vi "TCP IP Read Tester.vi"() -> ()   [LabVIEW 2015]
uses:
  Controls/QMH Fundamentals - Message Cluster.ctl
panel:
  in  "Test Read String":bool
  out "JSON Message":string="{\"PhoenixMsg\": {\n    \"Partition\" : \"EMP\",\n    \"Message\" : \"MSG\",\n    \"EnergyChannelId\" : 1,\n    \"IsActivated\" : True,\n    \"StopReason\" : 3,\n    \"Mode\" : 1,\n    \"PowerLevel\" : 32,\n}}"
  in  "Read":bool
  out "Cluster":T1
  out "Array":T2(array[cluster])
  in  "Fornax Executable Path":path=path "C:/Program Files (x86)/Medtronic/Fornax/x86/Fornax.exe"
  in  "error in (no error)":errorcluster
  out "Bipolar - Mode":string
  out "Bipolar - Power":string
  out "Mono2 Coag - Mode":string
  out "Mono2 Coag - Power":string
  out "Mono2 Cut - Mode":string
  out "Mono2 Cut - Power":string
  out "Mono1 Coag - Mode":string
  out "Mono1 Coag - Power":string
  out "Mono1 Cut - Mode":string
  out "Mono1 Cut - Power":string
  in  "Read String":string
  in  "stop":bool
  # "Mono1"
  # "Mono2"
  # "Bipolar"
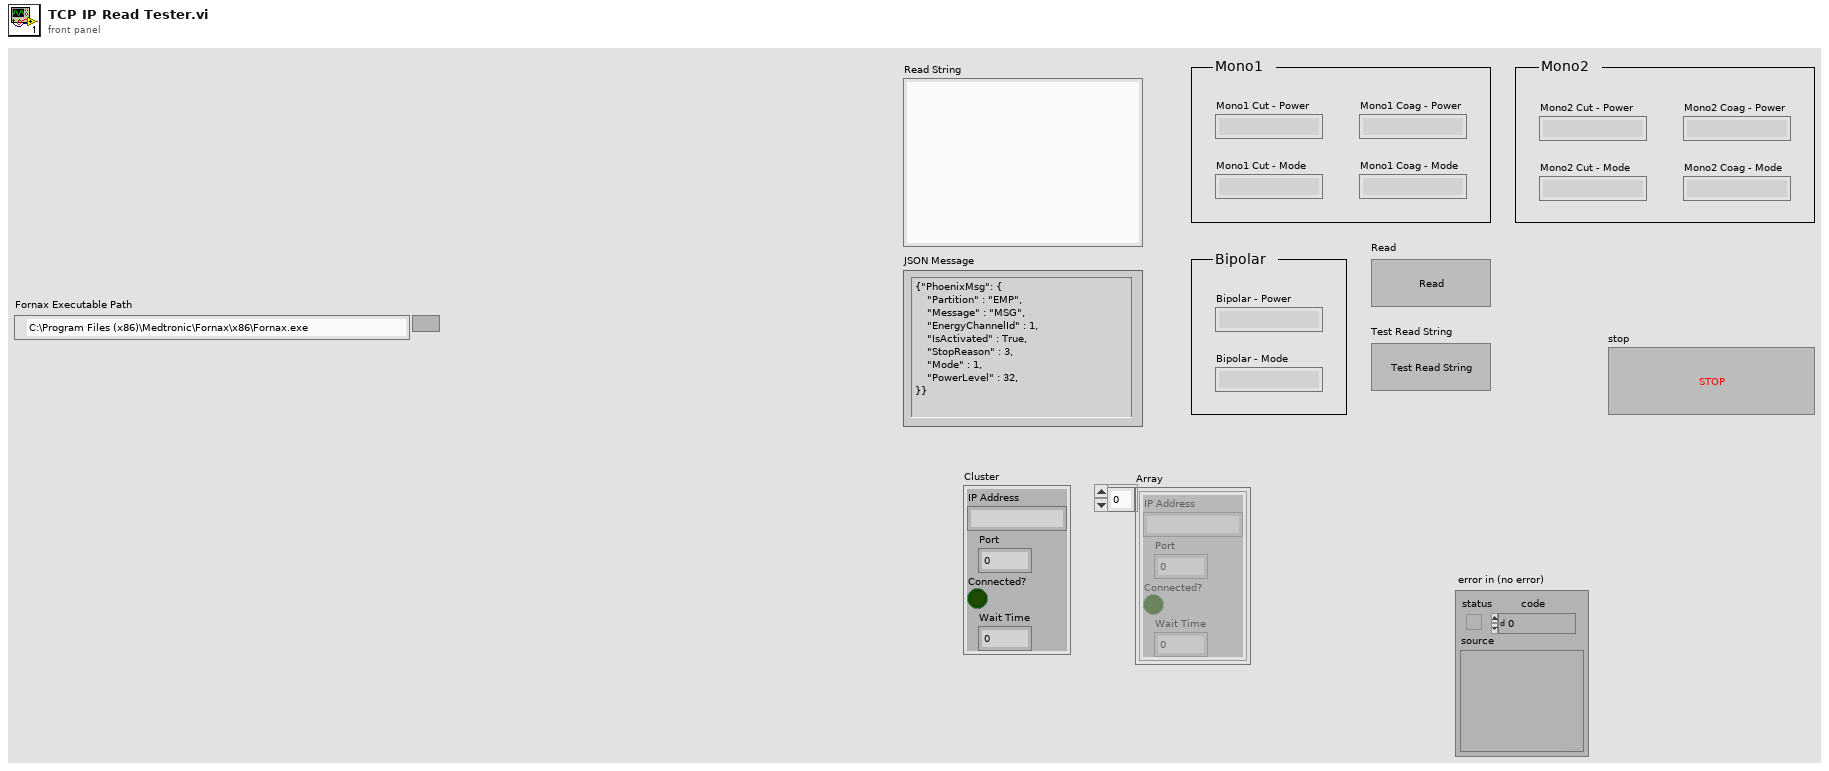
[diagram p1: front panel]
types:
  T1 = cluster{"IP Address":string, "Port":u16, "Connected?":bool, "Wait Time":dbl}
  T2 = cluster{"IP Address":string, "Port":u16, "Connected?":bool, "Wait Time":dbl}[]
  T3 = typedef "QMH Fundamentals - Message Cluster.ctl" = cluster{"Message":string, "Message Data":variant}
  T4 = cluster{"Mono1 Cut - Power":refnum<vi>, "Mono1 Cut - Mode":refnum<vi>, "Mono1 Coag - Power":refnum<vi>, "Mono1 Coag - Mode":refnum<vi>, "Mono2 Coag - Power":refnum<vi>, "Mono2 Coag - Mode":refnum<vi>, "Mono2 Cut - Power":refnum<vi>, "Mono2 Cut - Mode":refnum<vi>, "Bipolar - Power":refnum<vi>, "Bipolar - Mode":refnum<vi>}
  T5 = cluster{"Mono1 Cut Enum":refnum<vi>, "Mono1 - Cut Power":refnum<vi>, "Mono1 Coag Enum":refnum<vi>, "Mono1 - Coag Power":refnum<vi>, "Mono2 Cut Enum":refnum<vi>, "Mono2 - Cut Power":refnum<vi>, "Mono2 Coag Enum":refnum<vi>, "Mono2 - Coag Power":refnum<vi>, "Bipolar Enum":refnum<vi>, "Mono1 - Bipolar Power":refnum<vi>}
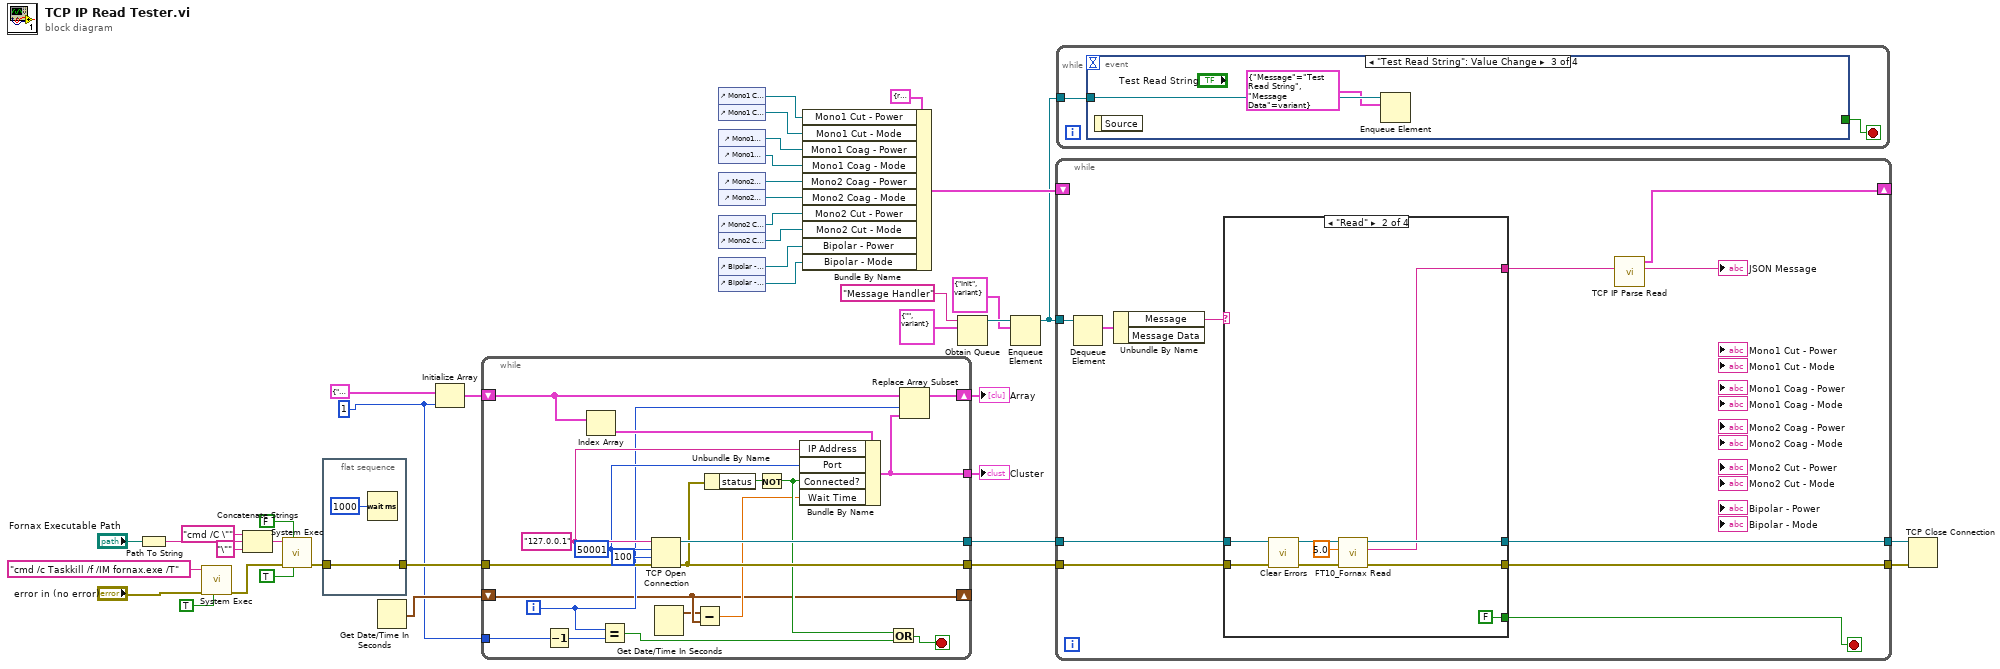
[diagram p0: block diagram]
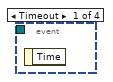
[diagram p2: hidden frame]
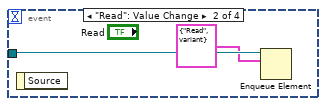
[diagram p3: hidden frame]
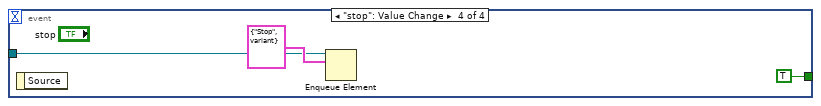
[diagram p4: hidden frame]
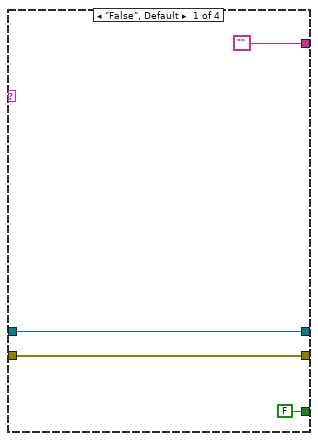
[diagram p5: hidden frame]
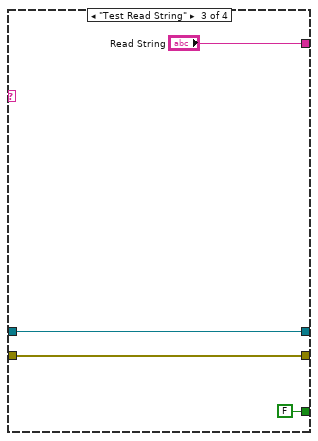
[diagram p6: hidden frame]
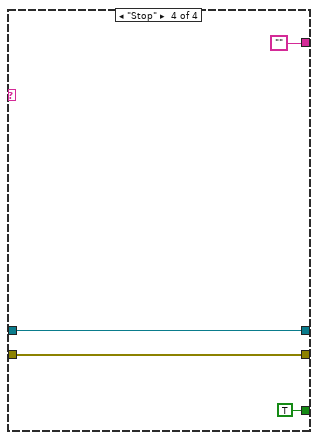
[diagram p7: hidden frame]
diagram:
  w12 = 1 ("dimension size")
  n1 = Path To String(path="Fornax Executable Path") -> (string=w18:string)
  n2 = call <vilib>:"System Exec.vi"("run minimized? (F)"=TRUE, "error in (no error)"="error in (no error)", "command line"="cmd /c Taskkill /f /IM fornax.exe /T") -> ("error out"=w24:errorcluster)  [unwired: 5 in, 3 out]
  n3 = Concatenate Strings("cmd /C \"" ("string"), w18, "\"" ("string")) -> (w20:string)
  n4 = call <vilib>:"System Exec.vi"("run minimized? (F)"=TRUE, "wait until completion? (T)"=FALSE, "error in (no error)"=w24, "command line"=w20) -> ("error out"=w15:errorcluster)  [unwired: 4 in, 3 out]
  n5 = flat-sequence {
    tunnel: [w42] -> w13
    tunnel: w15 -> [w42]
    frame #0 {
      n6 = Wait (ms)(milliseconds to wait=u32 1000) -> ()  [unwired: 1 out]
    }
  }
  n7 = Get Date/Time In Seconds() -> (seconds since 1Jan1904=w14:timestamp)
  n8 = Initialize Array(T1 {"IP Address"="", "Port"=0, "Connected?"=FALSE, "Wait Time"=0.0} ("Cluster"), w12) -> (w27:T2)
  n9 = while {
    tunnel: [w61] -> w9
    shift-right: [w60] -> w11
    shift-left: w27 -> [w59]
    tunnel: w12 -> [w50]
    tunnel: [w47] -> w10
    shift-right: [w44] -> _
    shift-left: w14 -> [w44]
    tunnel: w13 -> [w62]
    tunnel: [w55] -> w3
    i -> [w46]
    stop <- w52 stop-if-true
    w56 = u16 50001 ("remote port or service name")
    w57 = "127.0.0.1" ("address")
    n10 = Decrement(x=w50) -> (x-1=w49:i32)
    n11 = Index Array(array=w59) -> (element=w58:T1)  [unwired: 1 in]
    n12 = Equal?(x=w46, y=w49) -> (x = y?=w48:bool)
    n13 = TCP Open Connection(address=w57, remote port or service name=w56, timeout ms (60000)=100, error in (no error)=w62) -> (connection ID=w61:refnum<k5>, error out=w55:errorcluster)  [unwired: 1 in]
    n14 = Get Date/Time In Seconds() -> (seconds since 1Jan1904=w43:timestamp)
    n15 = Subtract(x=w43, y=w44) -> (x-y=w45:dbl)
    n16 = Unbundle By Name(w55) -> ("status"=w54:bool)
    n17 = Not(x=w54) -> (.not. x?=w51:bool)
    n18 = Bundle By Name(cluster=w58, "IP Address"=w57, "Port"=w56, "Connected?"=w51, "Wait Time"=w45) -> (w47:T1)
    n19 = Or(x=w51, y=w48) -> (x .or. y?=w52:bool)
    n20 = Replace Array Subset(array=w59, new element=w47, index=w46) -> (w60:T2)
  }
  "Array" <- w11
  "Cluster" <- w10
  n21 = control-ref of="Mono1 Cut - Power"() -> (w39:refnum<vi>)
  n22 = control-ref of="Mono1 Cut - Mode"() -> (w38:refnum<vi>)
  n23 = control-ref of="Mono1 Coag - Power"() -> (w37:refnum<vi>)
  n24 = control-ref of="Mono1 Coag - Mode"() -> (w36:refnum<vi>)
  n25 = control-ref of="Mono2 Coag - Power"() -> (w35:refnum<vi>)
  n26 = control-ref of="Mono2 Coag - Mode"() -> (w34:refnum<vi>)
  n27 = control-ref of="Mono2 Cut - Power"() -> (w33:refnum<vi>)
  n28 = control-ref of="Mono2 Cut - Mode"() -> (w32:refnum<vi>)
  n29 = control-ref of="Bipolar - Power"() -> (w31:refnum<vi>)
  n30 = control-ref of="Bipolar - Mode"() -> (w30:refnum<vi>)
  n31 = Bundle By Name(cluster=T4 {"Mono1 Cut - Power"=refnum, "Mono1 Cut - Mode"=refnum, "Mono1 Coag - Power"=refnum, "Mono1 Coag - Mode"=refnum, "Mono2 Coag - Power"=refnum, "Mono2 Coag - Mode"=refnum, "Mono2 Cut - Power"=refnum, "Mono2 Cut - Mode"=refnum, "Bipolar - Power"=refnum, "Bipolar - Mode"=refnum}, "Mono1 Cut - Power"=w39, "Mono1 Cut - Mode"=w38, "Mono1 Coag - Power"=w37, "Mono1 Coag - Mode"=w36, "Mono2 Coag - Power"=w35, "Mono2 Coag - Mode"=w34, "Mono2 Cut - Power"=w33, "Mono2 Cut - Mode"=w32, "Bipolar - Power"=w31, "Bipolar - Mode"=w30) -> (w29:T4)
  n32 = Obtain Queue(name (unnamed)="Message Handler", element data type=T3 {"Message"="", "Message Data"=variant} ("Message Cluster")) -> (queue out=w7:refnum<queue>)  [unwired: 3 in, 2 out]
  n33 = Enqueue Element(queue=w7, element=T3 {"Message"="Init", "Message Data"=variant}) -> (queue out=w4:refnum<queue>)  [unwired: 2 in, 2 out]
  n34 = while {
    shift-right: [w64] -> _
    shift-left: w29 -> [_]
    tunnel: w9 -> [w70]
    tunnel: w4 -> [w72]
    tunnel: w3 -> [w69]
    tunnel: [w68] -> w1
    tunnel: [w67] -> w2
    stop <- w63 stop-if-true
    n35 = Dequeue Element(queue=w72) -> (element=w73:T3)  [unwired: 2 in, 3 out]
    n36 = Unbundle By Name(w73) -> ("Message"=w71:string)  [unwired: 1 out]
    n37 = case shown="\"Read\"" w71 {
      tunnel: w70 -> [w77 w85 w88 w93]
      tunnel: w69 -> [w76 w83 w87 w92]
      tunnel: [w77 w82 w88 w93] -> w68
      tunnel: [w76 w81 w87 w92] -> w67
      tunnel: ["" w80 "Read String" ""] -> w66
      tunnel: [FALSE FALSE FALSE TRUE] -> w63
      frame "False", Default {
      }
      frame "Read" {
        n38 = call <vilib>:"Clear Errors.vi"("error in (no error)"=w83) -> ("error out"=w78:errorcluster)  [unwired: 5 in, 1 out]
        n39 = call "FT10_Fornax Read.vi"("error in (no error)"=w78, "Timeout"=5.0, "TCP Network Connection in"=w85) -> ("error out"=w81:errorcluster, "JSON Message"=w80:string, "TCP Network Connection out"=w82:refnum<k5>)  [unwired: 6 in]
      }
      frame "Test Read String" {
      }
      frame "Stop" {
      }
    }
    n40 = call "TCP IP Parse Read.vi"("JSON in"=w66) -> ("JSON out"=→"JSON Message":string, "Cluster out"=w64:T5)  [unwired: 9 in]
  }
  n41 = while {
    tunnel: w4 -> [w95]
    stop <- w94 stop-if-true
    n42 = event shown="[2] \"Test Read String\": Value Change" {
      selector: _ -> [_ _ _ _]
      dyn-events: _ -> [_ _ _ _]
      timeout: _ -> [_ _ _ _]
      tunnel: w95 -> [_ w97 w99 w101]
      tunnel: [_ _ _ TRUE] -> w94
      event Timeout {
        n43 = event-data() -> ()  [unwired: 1 in, 1 out]
      }
      event "Read": Value Change {
        n44 = event-data() -> ()  [unwired: 1 in, 1 out]
        n45 = Enqueue Element(queue=w97, element=T3 {"Message"="Read", "Message Data"=variant}) -> ()  [unwired: 2 in, 3 out]
      }
      event "Test Read String": Value Change {
        n46 = event-data() -> ()  [unwired: 1 in, 1 out]
        n47 = Enqueue Element(queue=w99, element=T3 {"Message"="Test Read String", "Message Data"=variant}) -> ()  [unwired: 2 in, 3 out]
      }
      event "stop": Value Change {
        n48 = event-data() -> ()  [unwired: 1 in, 1 out]
        n49 = Enqueue Element(queue=w101, element=T3 {"Message"="Stop", "Message Data"=variant}) -> ()  [unwired: 2 in, 3 out]
      }
    }
  }
  n50 = TCP Close Connection(connection ID=w1, error in (no error)=w2) -> ()  [unwired: 1 in, 2 out]
